vi "Button Prompt.vi"(7 "Timeout":i32, 8 "Error in":errorcluster caption="Error in (no error)", 10 "Button to Check":string(combo), 11 "TestRadio":refnum<class "SC Manufacturing Test.lvclass">) -> (0 "Error out":errorcluster, 3 "Pass":bool)   [LabVIEW 2015, in "Rocom Button Test.lvclass"]
uses:
  Rocom Button Test.lvclass
  Classes/Manufacturing Test/Class/SC Manufacturing Test.lvclass
panel:
  out "Done":bool
  out "DOWN":bool
  out "UP":bool
  out "OFF":bool
  out "ON":bool
  # "Button Press"
  # "Press and release\nthe flashing button."
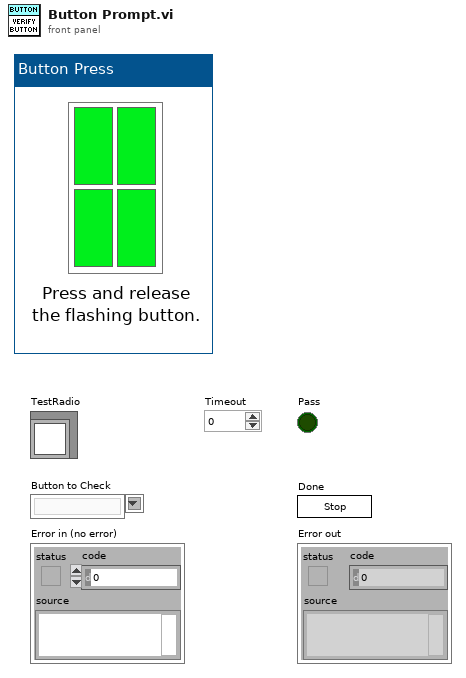
[diagram p1: front panel]
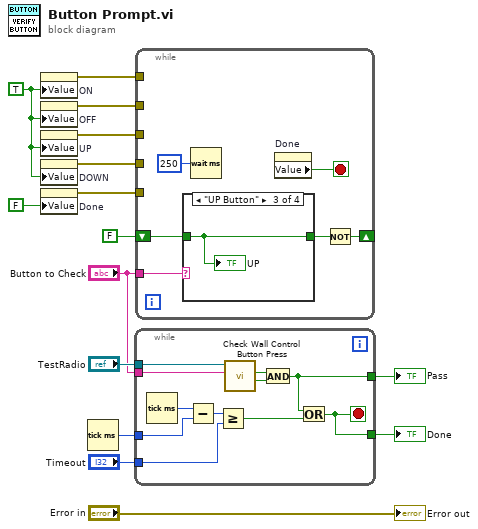
[diagram p0: block diagram]
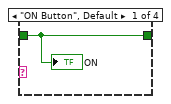
[diagram p2: hidden frame]
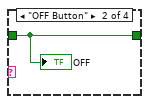
[diagram p3: hidden frame]
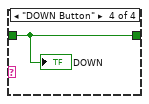
[diagram p4: hidden frame]
diagram:
  w14 = TRUE ("ON")
  n1 = property on="ON" class="Bool (strict)"("Value"=w14) -> (error out=w13:errorcluster)  [unwired: 2 in, 1 out]
  n2 = property on="OFF" class="Bool (strict)"("Value"=w14) -> (error out=w12:errorcluster)  [unwired: 2 in, 1 out]
  n3 = property on="UP" class="Bool (strict)"("Value"=w14) -> (error out=w11:errorcluster)  [unwired: 2 in, 1 out]
  n4 = property on="DOWN" class="Bool (strict)"("Value"=w14) -> (error out=w10:errorcluster)  [unwired: 2 in, 1 out]
  n5 = property on="Done" class="Bool (strict)"("Value"=FALSE ("ON")) -> (error out=w9:errorcluster)  [unwired: 2 in, 1 out]
  n6 = Tick Count (ms)() -> (millisecond timer value=w5:u32)
  n7 = while {
    tunnel: "TestRadio" -> [w24]
    tunnel: [w18] -> w6
    tunnel: w5 -> [w23]
    tunnel: "Timeout" -> [w20]
    tunnel: [w17] -> w3
    tunnel: "Button to Check" -> [w16]
    stop <- w17 stop-if-true
    n8 = Tick Count (ms)() -> (millisecond timer value=w22:u32)
    n9 = Subtract(x=w22, y=w23) -> (x-y=w21:u32)
    n10 = Greater Or Equal?(x=w21, y=w20) -> (x >= y?=w19:bool)
    n11 = call "Check Wall Control Button Press.vi"("Button to Check"=w16, "Acrobat Template in"=w24) -> ("Released"=w25:bool, "Pressed"=w26:bool)  [unwired: 6 in, 2 out]
    n12 = And(x=w26, y=w25) -> (x .and. y?=w18:bool)
    n13 = Or(x=w18, y=w19) -> (x .or. y?=w17:bool)
  }
  "Pass" <- w6
  "Done" <- w3
  n14 = while {
    tunnel: "Button to Check" -> [w31]
    shift-right: [w28] -> _
    shift-left: FALSE -> [w30]
    tunnel: w13 -> [_]
    tunnel: w12 -> [_]
    tunnel: w11 -> [_]
    tunnel: w10 -> [_]
    tunnel: w9 -> [_]
    stop <- w27 stop-if-true
    n15 = case shown="\"UP Button\"" w31 {
      tunnel: w30 -> [w33 w34 w35 w36]
      tunnel: [w33 w34 w35 w36] -> w29
      frame "ON Button", Default {
        "ON" <- w33
      }
      frame "OFF Button" {
        "OFF" <- w34
      }
      frame "UP Button" {
        "UP" <- w35
      }
      frame "DOWN Button" {
        "DOWN" <- w36
      }
    }
    n16 = Wait (ms)(milliseconds to wait=u32 250) -> ()  [unwired: 1 out]
    n17 = property on="Done" class="Bool (strict)"() -> ("Value"=w27:bool)  [unwired: 2 in, 2 out]
    n18 = Not(x=w29) -> (.not. x?=w28:bool)
  }
  "Error out" <- "Error in"
